vi "Handle GroupData.vi"(7 "Source ID":u32, 8 "GroupData":T1, 9 "Sequence":u32, 10 "ChannelService":refnum<class "ChannelService.lvclass">, 11 "Subscription Loop Data in":T2) -> (0 "error out":errorcluster, 3 "Subscription Loop Data":T2)   [LabVIEW 2020, in "Vecto.lvlib" / "RemoteDataService.lvclass"]
uses:
  RemoteDataService.lvclass
  Subscription Loop Data.ctl
  Subscription Group Info.ctl
  proto/GroupData/Data.ctl
  ChannelService/ChannelService.lvclass
  <vilib>/Utility/miscctls.llb/LVMapReplaceAction.ctl
  RemoteDataService.lvclass/RemoteDataService.ctl
  Group/Group.lvclass
  proto/GroupData/GroupData.lvlib
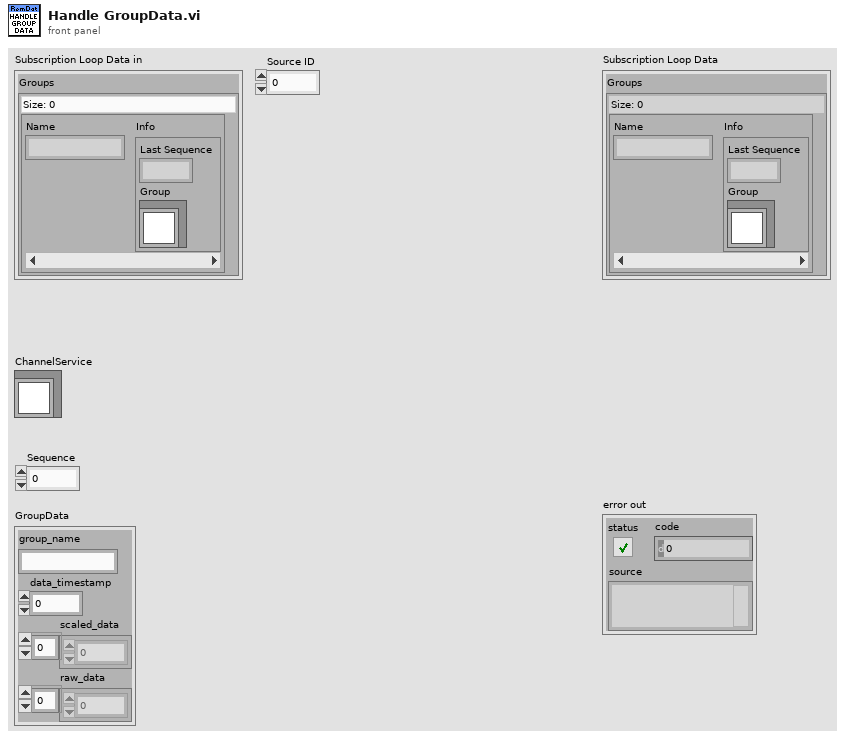
[diagram p1: front panel]
types:
  T1 = typedef "GroupData.lvlib/Data.ctl" = cluster{"group_name":string, "data_timestamp":i64, "scaled_data":dbl[], "raw_data":dbl[]}
  T2 = typedef "Vecto.lvlib/RemoteDataService.lvclass/Subscription Loop Data.ctl" = cluster{"Groups":map{string, T3}}
  T3 = typedef "Vecto.lvlib/RemoteDataService.lvclass/Subscription Group Info.ctl" = cluster{"Last Sequence":u32, "Group":refnum<class "Group.lvclass">}
  T4 = typedef "LVMapReplaceAction.ctl" = enum32{"Modify Entry only if found", "Add or Modify Entry", "Delete Entry"}
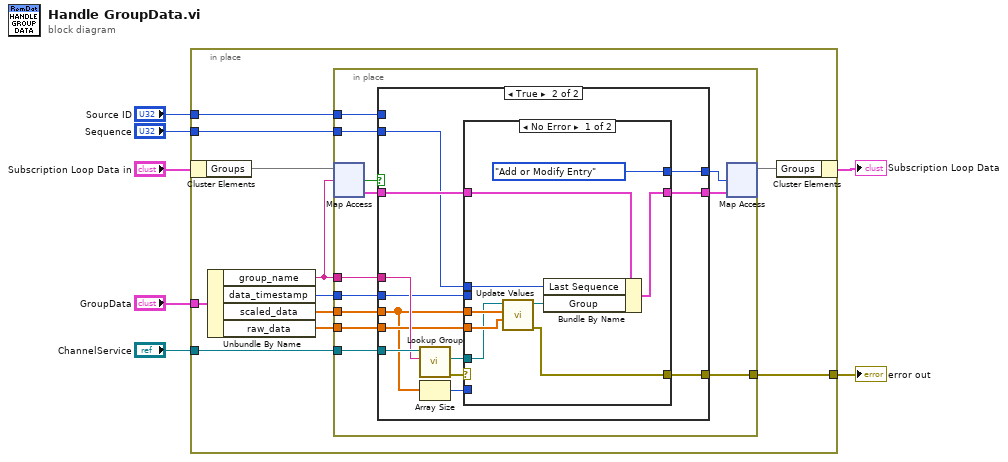
[diagram p0: block diagram]
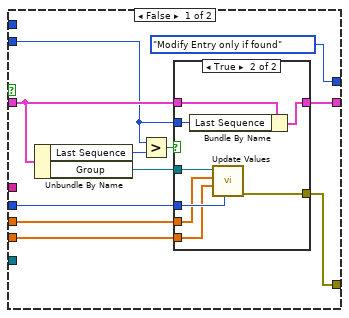
[diagram p2: hidden frame]
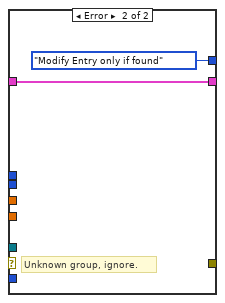
[diagram p4: hidden frame]
diagram:
  n1 = in-place {
    in-place-border: "GroupData" -> [w8]
    in-place-border: "ChannelService" -> [w17]
    in-place-border: "Sequence" -> [w12]
    in-place-border: "Source ID" -> [w11]
    in-place-border: [w9] -> w2
    n2 = in-place-cluster #1("Subscription Loop Data in") -> ("Groups"=w18:map{string, T3})
    n3 = Unbundle By Name(w8) -> ("group_name"=w16:string, "data_timestamp"=w13:i64, "scaled_data"=w14:dbl[], "raw_data"=w15:dbl[])
    n4 = in-place {
      in-place-border: w17 -> [w28]
      in-place-border: w16 -> [w27]
      in-place-border: w15 -> [w26]
      in-place-border: w14 -> [w25]
      in-place-border: w13 -> [w24]
      in-place-border: w12 -> [w23]
      in-place-border: w11 -> [w22]
      in-place-border: [w20] -> w9
      n5 = in-place-map #2(w18, w16) -> (w29:T3, w30:bool)  [unwired: 1 in]
      n6 = case shown="True" w30 {
        tunnel: w29 -> [w35 w58]
        tunnel: w28 -> [_ w63]
        tunnel: w27 -> [_ w61]
        tunnel: w26 -> [w36 w55]
        tunnel: w25 -> [w37 w54]
        tunnel: w24 -> [w38 w56]
        tunnel: w23 -> [w33 w57]
        tunnel: w22 -> [_ _]
        tunnel: [w34 w53] -> w21
        tunnel: [w32 w52] -> w20
        tunnel: [LVMapReplaceAction."Modify Entry only if found" ("action") w51] -> w19
        frame False {
          n7 = Unbundle By Name(w35) -> ("Last Sequence"=w41:u32, "Group"=w40:refnum<class "Group.lvclass">)
          n8 = Greater?(x=w33, y=w41) -> (0:w39:bool)
          n9 = case shown="True" w39 {
            tunnel: w40 -> [_ w50]
            tunnel: w38 -> [_ w49]
            tunnel: w37 -> [_ w48]
            tunnel: w36 -> [_ w47]
            tunnel: w35 -> [w42 w46]
            tunnel: [w42 w44] -> w34
            tunnel: w33 -> [_ w45]
            tunnel: [_ w43] -> w32
            frame False {
              # "Older data, ignore"
            }
            frame True {
              n10 = Bundle By Name(cluster=w46, "Last Sequence"=w45) -> (w44:T3)
              n11 = call "Update Values.vi"("Timestamp (Now)"=w49, "Raw Values (N/A)"=w47, "Values"=w48, "Group in"=w50) -> ("error out"=w43:errorcluster)  [unwired: 6 in, 1 out]
            }
          }
        }
        frame True {
          n12 = call "Lookup Group.vi"("Group Name"=w61, "ChannelService in"=w63) -> ("error out"=w62:errorcluster, "Group"=w60:refnum<class "Group.lvclass">)  [unwired: 7 in, 1 out]
          n13 = Array Size(array=w54) -> (size(s)=w59:i32)
          n14 = case shown="No Error" w62 {
            tunnel: w60 -> [w64 _]
            tunnel: w59 -> [_ _]
            tunnel: w58 -> [w72 w73]
            tunnel: w57 -> [w71 _]
            tunnel: w56 -> [_ _]
            tunnel: w55 -> [w70 _]
            tunnel: w54 -> [w69 _]
            tunnel: [w68 w73] -> w53
            tunnel: [w67 _] -> w52
            tunnel: [LVMapReplaceAction."Add or Modify Entry" ("action") LVMapReplaceAction."Modify Entry only if found" ("action")] -> w51
            frame No Error {
              n15 = call "Update Values.vi"("Raw Values (N/A)"=w70, "Values"=w69, "Group in"=w64) -> ("error out"=w67:errorcluster, "Group out"=w66:refnum<class "Group.lvclass">)  [unwired: 7 in]
              n16 = Bundle By Name(cluster=w72, "Last Sequence"=w71, "Group"=w66) -> (w68:T3)
            }
            frame Error {
              # "Unknown group, ignore."
            }
          }
        }
      }
      n17 = in-place-map #2(w21, w19) -> (w10:map{string, T3})  [unwired: 2 out]
    }
    n18 = in-place-cluster #1("Groups"=w10) -> (→"Subscription Loop Data":T2)
  }
  "error out" <- w2
